vi "Repeat Until Timeout.vi"(7 "Name":string="Repeat Until Timeout", 8 "On Timeout Status":T1, 9 "Timeout (s)":dbl, 10 "Finish On":T2, 11 "Node In":refnum<class "abs_Node.lvclass">) -> (3 "Node Out":refnum<class "abs_Node.lvclass">)   [LabVIEW 2021, in "BT.lvlib"]
uses:
  BT.lvlib
  abs_Node/abs_Node.lvclass
  Repeater/Support/Finish On - Type.ctl
  Repeat Until Timeout/Support/On Timeout Status - Type.ctl
  Repeat Until Timeout/Repeat Until Timeout.lvclass
  C:/Users/Tim/Documents/LabVIEW/2021/Behaviour Tree/abs_Node/abs_Node.lvclass
  C:/Users/Tim/Documents/LabVIEW/2021/Behaviour Tree/abs_Decorator/abs_Decorator.lvclass
  C:/Users/Tim/Documents/LabVIEW/2021/Behaviour Tree/Repeater/Repeater.lvclass
  abs_Node/abs_Node.lvclass/abs_Node.ctl
  abs_Decorator/abs_Decorator.lvclass/abs_Decorator.ctl
  Repeater/Repeater.lvclass/Repeater.ctl
  Repeat Until Timeout/Repeat Until Timeout.lvclass/Repeat Until Timeout.ctl
  abs_Node/Properties/Write Name.vi
  abs_Decorator/Properties/Write Node.vi
  Repeater/Properties/Write Finish On.vi
  Repeat Until Timeout/Properties/Write On Timeout Status.vi
  Repeat Until Timeout/Properties/Write Timeout.vi
  Repeater/Repeater.lvclass
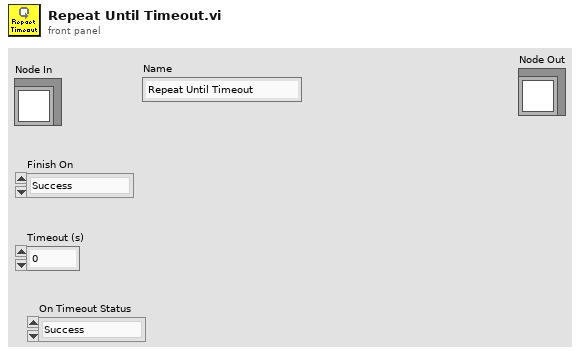
[diagram p1: front panel]
types:
  T1 = typedef "BT.lvlib/Repeat Until Timeout.lvclass/On Timeout Status - Type.ctl" = enum16{"Success", "Failure"}
  T2 = typedef "BT.lvlib/Repeater.lvclass/Finish On - Type.ctl" = enum16{"Success", "Failure", "Never"}
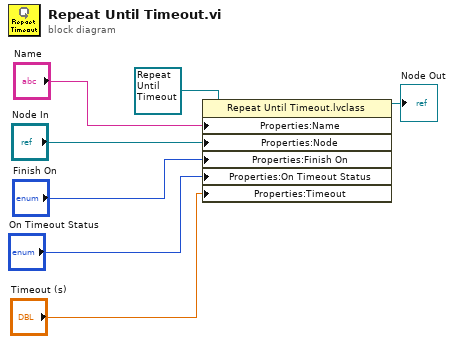
[diagram p0: block diagram]
diagram:
  n1 = property class="Repeat Until Timeout.lvclass"(reference=refnum<class "Repeat Until Timeout.lvclass"> refnum ("BT.lvlib:Repeat Until Timeout.lvclass"), "Properties:Name"="Name", "Properties:Node"="Node In", "Properties:Finish On"="Finish On", "Properties:On Timeout Status"="On Timeout Status", "Properties:Timeout"="Timeout (s)") -> (reference out=→"Node Out":refnum<class "Repeat Until Timeout.lvclass">)  [unwired: 1 in, 1 out]
